vi "boolean-string converter.vi"(2 "Boolean in":bool, 4 "string in":string) -> (0 "string out":string, 1 "Boolean out":bool)   [LabVIEW 2015]
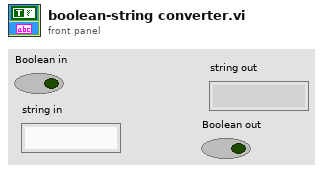
[diagram p1: front panel]
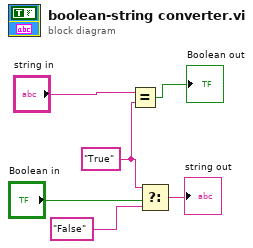
[diagram p0: block diagram]
diagram:
  w2 = "True"
  n1 = Equal?(x="string in", y=w2) -> (x = y?=→"Boolean out":bool)
  n2 = Select(t=w2, s="Boolean in", f="False") -> (s? t:f=→"string out":string)
